vi "SwitchBoard_init.vi"(8 "error in":errorcluster) -> (0 "error out":errorcluster, 3 "Handle":u32)   [LabVIEW 2016]
panel:
  in  "Flow Control":u16(ring) items=["None"=0, "RTS-CTS"=256, "DTR-DSR"=512, "XOn-XOff"=1024]
  in  "Word Length":u8(ring)=8 items=["FT_BITS_7"=7, "FT_BITS_8"=8]
  in  "Stop Bits":u8(ring) items=["FT_STOP_BITS_1"=0, "FT_STOP_BITS_2"=2]
  in  "Parity":u8(ring) items=["FT_PARITY_NONE", "FT_PARITY_ODD", "FT_PARITY_EVEN", "FT_PARITY_MARK", "FT_PARITY_SPACE"]
  in  "Baud Rate":u32=115200
  in  "Device Index":u32
  out "Device Description":string
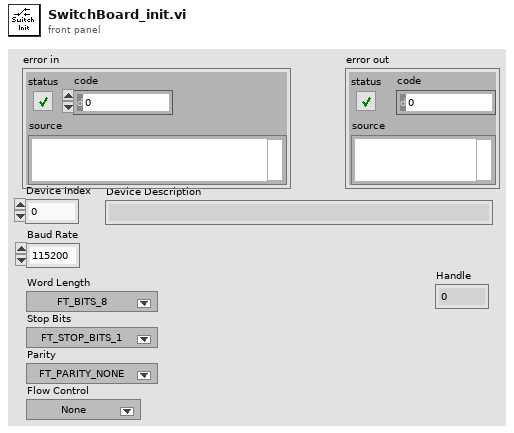
[diagram p1: front panel]
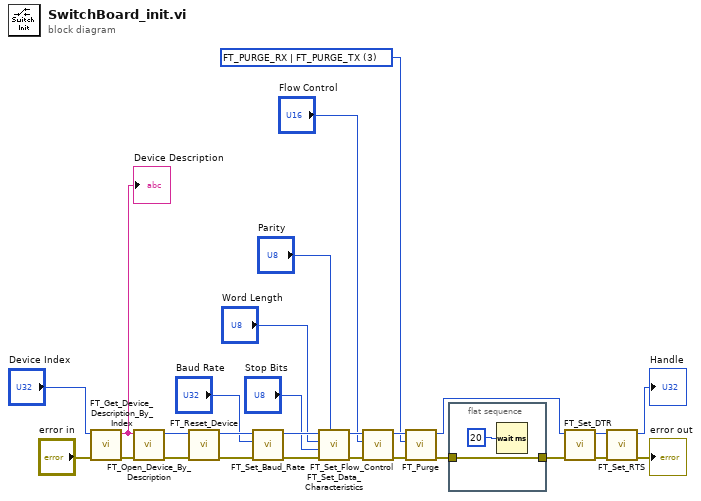
[diagram p0: block diagram]
diagram:
  w3 = u32 3 items=["FT_PURGE_RX"=1, "FT_PURGE_TX"=2, "FT_PURGE_RX | FT_PURGE_TX"=3] ("Purge Flags")
  n1 = call <instrlib>:"FT_Get_Device_Description_By_Index.vi"("error in"="error in", "Device Index"="Device Index") -> ("error out"=w24:errorcluster, "Device Description"=w27:string)  [unwired: 8 in]
  "Device Description" <- w27
  n2 = call <instrlib>:"FT_Open_Device_By_Description.vi"("error in"=w24, "Device Description"=w27) -> ("error out"=w23:errorcluster, "Handle"=w26:u32)  [unwired: 8 in]
  n3 = call <instrlib>:"FT_Reset_Device.vi"("error in"=w23, "Handle"=w26) -> ("error out"=w21:errorcluster, "Handle out"=w22:u32)  [unwired: 8 in]
  n4 = call <instrlib>:"FT_Set_Baud_Rate.vi"("error in"=w21, "Baud Rate"="Baud Rate", "Handle"=w22) -> ("error out"=w20:errorcluster, "Handle out"=w19:u32)  [unwired: 7 in]
  n5 = call <instrlib>:"FT_Set_Data_Characteristics.vi"("Parity"="Parity", "error in"=w20, "Stop Bits"="Stop Bits", "Word Length"="Word Length", "Handle"=w19) -> ("error out"=w18:errorcluster, "Handle out"=w17:u32)  [unwired: 5 in]
  n6 = call <instrlib>:"FT_Set_Flow_Control.vi"("error in"=w18, "Flow Control"="Flow Control", "Handle"=w17) -> ("error out"=w16:errorcluster, "Handle out"=w15:u32)  [unwired: 7 in]
  n7 = call <instrlib>:"FT_Purge.vi"("error in"=w16, "Purge Flags"=w3, "Handle"=w15) -> ("error out"=w2:errorcluster, "Handle out"=w14:u32)  [unwired: 7 in]
  n8 = flat-sequence {
    tunnel: w2 -> [w28]
    tunnel: [w28] -> w1
    frame #0 {
      n9 = Wait (ms)(milliseconds to wait=u32 20) -> ()  [unwired: 1 out]
    }
  }
  n10 = call <instrlib>:"FT_Set_DTR.vi"("error in"=w1, "Handle"=w14) -> ("error out"=w12:errorcluster, "Handle out"=w13:u32)  [unwired: 8 in]
  n11 = call <instrlib>:"FT_Set_RTS.vi"("error in"=w12, "Handle"=w13) -> ("error out"=→"error out":errorcluster, "Handle out"=→"Handle":u32)  [unwired: 8 in]
